vi "CreateProduct.vi"(8 "error in (no error)":errorcluster, 11 "CreatorB":refnum<class "CreatorB.lvclass">) -> (0 "error out":errorcluster, 2 "Product":refnum<class "Product.lvclass">, 3 "CreatorB":refnum<class "CreatorB.lvclass">)   [LabVIEW 2020, in "FactoryMethod.lvlib" / "FactoryMethodLazyEvaluation.lvlib" / "CreatorB.lvclass"]
uses:
  CreatorB.lvclass
  Product/Product.lvclass
  ProductB/ProductB.lvclass
  E:/Francesco/GitHub/Design-Patterns-GoF_-_NI-LV/Creational/FactoryMethod/GoF_Example/FactoryMethodLazyEvaluation/Product/Product.lvclass
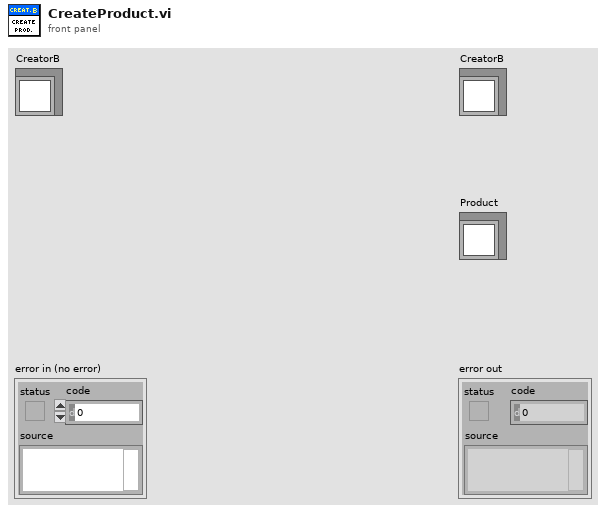
[diagram p1: front panel]
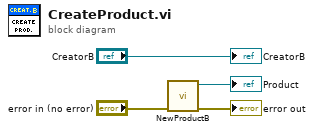
[diagram p0: block diagram]
diagram:
  n1 = call "NewProductB.vi"("error in (no error)"="error in (no error)") -> ("error out"=→"error out":errorcluster, "ProductB"=→"Product":refnum<class "ProductB.lvclass">)  [unwired: 9 in]
  "CreatorB" <- "CreatorB"
